vi "Experiment header-Save_Load AOL Z section.vi"(6 "AOL z-stack duration (sec)":dbl, 8 "error in (no error)":errorcluster, 9 "Function":enum16{"Write", "Read"}(ring)) -> (0 "error out":errorcluster)   [LabVIEW 2020]
uses:
  <vilib>/Utility/config.llb/Write Key (Double).vi
  <vilib>/Utility/config.llb/NI_LVConfig.lvlib
  <vilib>/Utility/config.llb/Write Key (Boolean).vi
  <vilib>/Utility/config.llb/Write Key (String).vi
  <vilib>/Utility/config.llb/Read Key (Boolean).vi
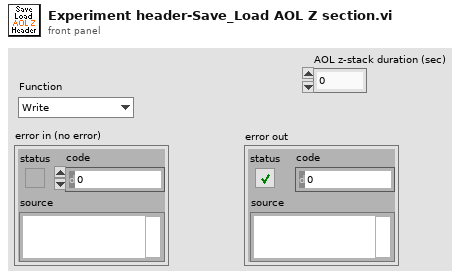
[diagram p1: front panel]
types:
  T1 = typedef "Fixed strings.ctl" = cluster{"ROI file name":string, "Normalised ROI file name":string, "Zplane Pockels values file name":string, "Functional data folder name":string, "Experiment Header file name":string, "Z-stack images folder name":string, "Groups setup rel. path":string, "Groups text file rel. path":string, "TDMS files folder name (F.img)":string, "TDMS files folder name (V.acq)":string, "TDMS files folder name (Pl.acq)":string, "Cycle rel times sequence file":string, "Dynamically called VIs folder name":string, "Time Series folder base name":string}
  T2 = typedef "NI_LVConfig.lvlib/Config Data RefNum.ctl" = refnum<k1>
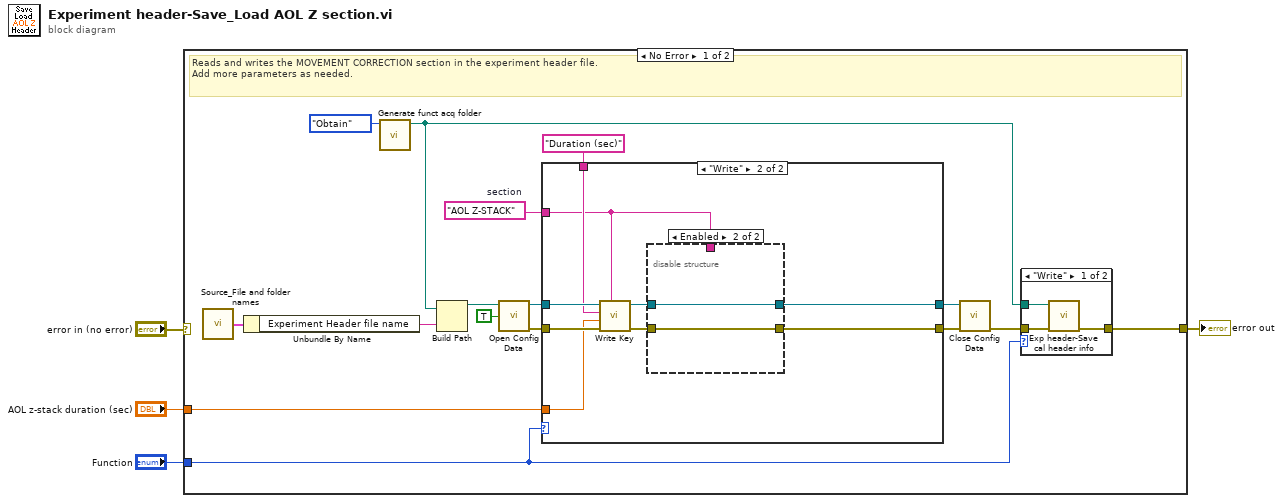
[diagram p0: block diagram]
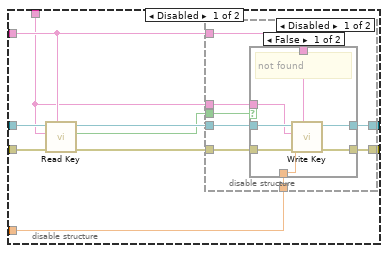
[diagram p4: hidden frame]
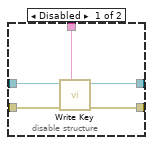
[diagram p7: hidden frame]
diagram:
  n1 = case shown="No Error" "error in (no error)" {
    selector: "error in (no error)" -> [_ w80]
    tunnel: [w13 w80] -> w4
    tunnel: "Function" -> [w12 _]
    tunnel: "AOL z-stack duration (sec)" -> [w15 _]
    frame No Error {
      w19 = "AOL Z-STACK"  # section
      # "Reads and writes the MOVEMENT CORRECTION section in the experiment header file.\nAdd more parameters as needed."
      n2 = call "Source_File and folder names.vi"() -> ("Fixed strings"=w8:T1)  [unwired: 1 in]
      n3 = Unbundle By Name(w8) -> ("Experiment Header file name"=w9:string)
      n4 = call "Generate funct acq folder.vi"("Function"=enum16{"Generate", "Obtain"}."Obtain") -> ("Funct acq experiment folder path"=w5:path)  [unwired: 9 in, 1 out]
      n5 = Build Path(base path=w5, name or relative path=w9) -> (appended path=w10:path)
      n6 = call <vilib>:"Open Config Data.vi"("create file if necessary (T)"=TRUE, "configuration file path"=w10) -> ("error out"=w18:errorcluster, "refnum"=w16:T2)  [unwired: 7 in, 1 out]
      n7 = case shown="\"Write\"" w12 {
        tunnel: w16 -> [w31 w71]
        tunnel: [w29 w65] -> w7
        tunnel: [w28 w64] -> w17
        tunnel: w18 -> [w30 w70]
        tunnel: w19 -> [w27 w63]
        tunnel: "Duration (sec)" ("key") -> [w26 w69]
        tunnel: w15 -> [w25 w68]
        frame "Read" {
          n8 = disable-structure shown="Enabled" {
            disable-tunnel: w31 -> [w41 w62]
            disable-tunnel: w30 -> [w40 w61]
            disable-tunnel: [w37 w62] -> w29
            disable-tunnel: [w36 w61] -> w28
            disable-tunnel: w27 -> [w35 _]
            disable-tunnel: w26 -> [w34 _]
            disable-tunnel: w25 -> [w33 _]
            frame Disabled {
              n9 = call-poly <vilib>:"Read Key.vi"("section"=w35, "error in (no error)"=w40, "key"=w34, "refnum"=w41) -> ("error out"=w38:errorcluster, "found?"=w32:bool, "refnum out"=w39:T2)  [unwired: 4 in, 1 out]
              n10 = disable-structure shown="Disabled" {
                disable-tunnel: w39 -> [w49 w60]
                disable-tunnel: w38 -> [w48 w59]
                disable-tunnel: [w47 w60] -> w37
                disable-tunnel: [w46 w59] -> w36
                disable-tunnel: w35 -> [w45 _]
                disable-tunnel: w34 -> [w44 _]
                disable-tunnel: w33 -> [w43 _]
                disable-tunnel: w32 -> [w42 _]
                frame Disabled {
                  n11 = case shown="False" w42 {
                    tunnel: w49 -> [w56 w58]
                    tunnel: w48 -> [w55 w57]
                    tunnel: [w54 w58] -> w47
                    tunnel: [w53 w57] -> w46
                    tunnel: w45 -> [w52 _]
                    tunnel: w44 -> [w51 _]
                    tunnel: w43 -> [w50 _]
                    frame False {
                      # "not found"
                      n12 = call-poly <vilib>:"Write Key.vi"("section"=w52, "error in (no error)"=w55, "value"=w50, "key"=w51, "refnum"=w56) -> ("error out"=w53:errorcluster, "refnum out"=w54:T2)  [unwired: 4 in, 1 out]
                    }
                    frame True {
                      # "found"
                    }
                  }
                }
                frame Enabled {
                }
              }
            }
            frame Enabled {
            }
          }
        }
        frame "Write" {
          n13 = call-poly <vilib>:"Write Key.vi"("section"=w63, "error in (no error)"=w70, "value"=w68, "key"=w69, "refnum"=w71) -> ("error out"=w66:errorcluster, "refnum out"=w67:T2)  [unwired: 4 in, 1 out]
          n14 = disable-structure shown="Enabled" {
            disable-tunnel: w67 -> [w77 w79]
            disable-tunnel: w66 -> [w76 w78]
            disable-tunnel: [w75 w79] -> w65
            disable-tunnel: [w74 w78] -> w64
            disable-tunnel: w63 -> [w73 _]
            frame Disabled {
              n15 = call-poly <vilib>:"Write Key.vi"("section"=w73, "error in (no error)"=w76, "refnum"=w77) -> ("error out"=w74:errorcluster, "refnum out"=w75:T2, "key"=w72:string)  [unwired: 5 in, 1 out]
            }
            frame Enabled {
            }
          }
        }
      }
      n16 = call <vilib>:"Close Config Data.vi"("error in (no error)"=w17, "refnum"=w7) -> ("error out"=w14:errorcluster)  [unwired: 8 in, 1 out]
      n17 = case shown="\"Write\"" w12 {
        tunnel: w14 -> [w23 w24]
        tunnel: [w22 w24] -> w13
        tunnel: w5 -> [w21 _]
        frame "Write" {
          n18 = call "Exp header-Save cal header info.vi"("error in (no error)"=w23, "Experiment folder path"=w21) -> ("error out"=w22:errorcluster)  [unwired: 9 in]
        }
        frame "Read", Default {
        }
      }
    }
    frame Error {
    }
  }
  "error out" <- w4
